vi "ReadI2C.vi"(6 "Timeout (1000ms)":u16=1000, 8 "error in (no error)":errorcluster, 10 "Bytes to Read":u8=1, 11 "GrovePi in":refnum<class "GrovePi.lvclass">) -> (0 "error out":errorcluster, 2 "Message":u8[](array[numeric]) format="%.0x", 3 "GrovePi out":refnum<class "GrovePi.lvclass">)   [LabVIEW 2014, in "GrovePi.lvclass"]
doc: "Reads a response back from the GrovePi over the I2C bus."
uses:
  GrovePi.lvclass
  GrovePi.lvclass/GrovePi.ctl
  I2C/I2C.lvclass
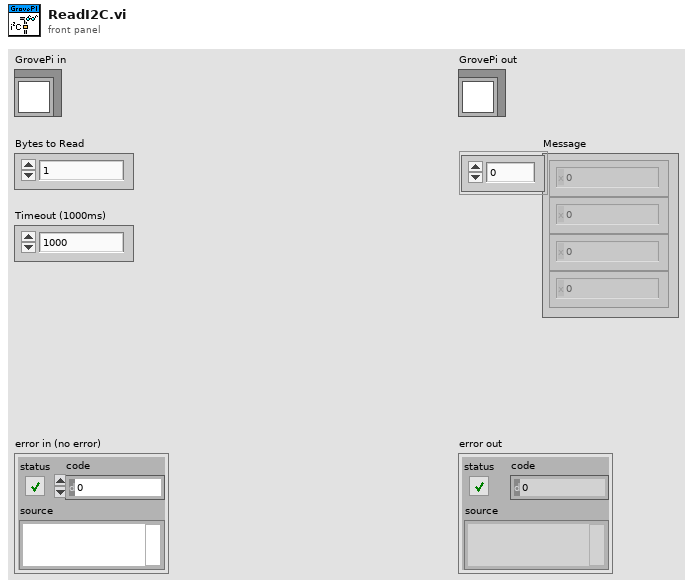
[diagram p1: front panel]
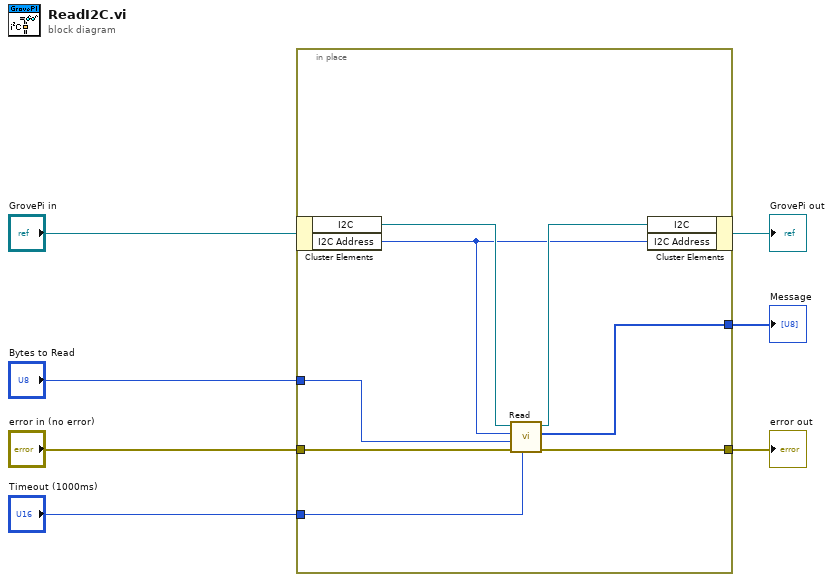
[diagram p0: block diagram]
diagram:
  n1 = in-place {
    in-place-border: "error in (no error)" -> [w15]
    in-place-border: [w11] -> w3
    in-place-border: [w10] -> w6
    in-place-border: "Bytes to Read" -> [w9]
    in-place-border: "Timeout (1000ms)" -> [w8]
    n2 = in-place-cluster #1("GrovePi in") -> ("I2C"=w14:refnum<class "I2C.lvclass">, "I2C Address"=w12:u8)
    n3 = call-dynamic "Read.vi"("Timeout (1000 ms)"=w8, "error in (no error)"=w15, "Bytes to Read"=w9, "I2C Slave Address"=w12, "I2C in"=w14) -> ("error out"=w11:errorcluster, "Data"=w10:u8[], "I2C out"=w13:refnum<class "I2C.lvclass">)  [unwired: 4 in]
    n4 = in-place-cluster #1("I2C"=w13, "I2C Address"=w12) -> (→"GrovePi out":refnum<class "GrovePi.lvclass">)
  }
  "Message" <- w6
  "error out" <- w3
